vi "Insight String Package.vi"(1 "Footer":string, 2 "String":string, 3 "Header":string) -> (0 "resulting string":string)   [LabVIEW 2012]
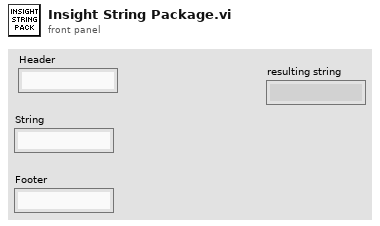
[diagram p1: front panel]
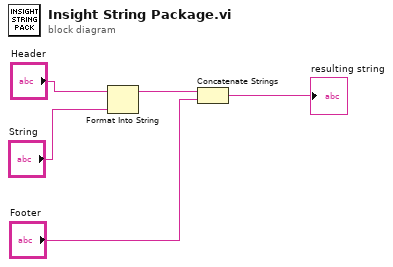
[diagram p0: block diagram]
diagram:
  n1 = Format Into String(initial string="Header", "String") -> (resulting string=w2:string)  [unwired: 2 in, 1 out]
  n2 = Concatenate Strings(w2, "Footer") -> (→"resulting string":string)
